vi "Bank With Semaphore.vi"() -> ()   [LabVIEW 2010]
doc: "This VI is a solution to the exercise in LabVIEW Core I that demonstrates race conditions. Without protecting critical code, as done here with semaphores, this VI could lose either a withdrawal or a deposit if done simultaneously."
panel:
  out "Balance":dbl
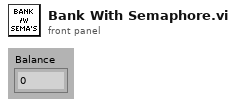
[diagram p1: front panel]
types:
  T1 = typedef "Account Info.ctl" = cluster{"Bank Rendezvous":T2, "Withdrawal Queue":refnum<queue>, "Deposit Queue":refnum<queue>}
  T2 = typedef "Rendezvous RefNum" = refnum<k1>
  T3 = typedef "Semaphore RefNum" = refnum<k1>
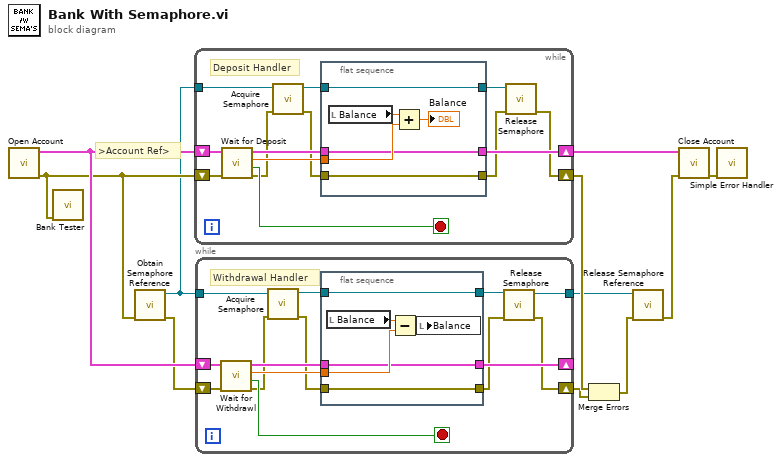
[diagram p0: block diagram]
diagram:
  # ">Account Ref>"
  n1 = call "Open Account.vi"() -> ("error out"=w6:errorcluster, "Account info"=w11:T1)  [unwired: 10 in]
  n2 = call "Bank Tester.vi"("error in (no error)"=w6) -> ()  [unwired: 10 in, 1 out]
  n3 = call <vilib>:"Obtain Semaphore Reference.vi"("error in (no error)"=w6) -> ("error out"=w5:errorcluster, "semaphore"=w1:T3)  [unwired: 4 in, 1 out]
  n4 = while {
    shift-right: [w20] -> w8
    shift-left: w11 -> [w23]
    shift-right: [w12] -> w10
    shift-left: w6 -> [w22]
    tunnel: w1 -> [w16]
    stop <- w19 stop-if-true
    # "Deposit Handler"
    n5 = call "Wait for Deposit.vi"("error in (no error)"=w22, "Account info"=w23) -> ("error out"=w15:errorcluster, "Stop?"=w19:bool, "Deposit Amount"=w24:dbl, "Account info out"=w21:T1)  [unwired: 6 in]
    n6 = call <vilib>:"Acquire Semaphore.vi"("error in (no error)"=w15, "semaphore"=w16) -> ("error out"=w14:errorcluster, "semaphore out"=w17:T3)  [unwired: 3 in, 1 out]
    n7 = flat-sequence {
      tunnel: w24 -> [w30]
      tunnel: [w27] -> w20
      tunnel: w21 -> [w27]
      tunnel: w14 -> [w26]
      tunnel: [w26] -> w13
      tunnel: [w25] -> w18
      tunnel: w17 -> [w25]
      frame #0 {
        n8 = local read "Balance"() -> (w28:dbl)
        n9 = Add(x=w28, y=w30) -> (x+y=→"Balance":dbl)
      }
    }
    n10 = call <vilib>:"Release Semaphore.vi"("error in (no error)"=w13, "semaphore"=w18) -> ("error out"=w12:errorcluster)  [unwired: 4 in, 1 out]
  }
  n11 = while {
    shift-right: [w40] -> _
    shift-left: w11 -> [w43]
    shift-right: [w31] -> w9
    shift-left: w5 -> [w42]
    tunnel: w1 -> [w38]
    tunnel: [w35] -> w4
    stop <- w39 stop-if-true
    # "Withdrawal Handler"
    n12 = call "Wait for Withdrawl.vi"("error in (no error)"=w42, "Account info"=w43) -> ("error out"=w34:errorcluster, "Stop?"=w39:bool, "Withdrawal Amount"=w44:dbl, "Account info out"=w41:T1)  [unwired: 6 in]
    n13 = call <vilib>:"Acquire Semaphore.vi"("error in (no error)"=w34, "semaphore"=w38) -> ("error out"=w33:errorcluster, "semaphore out"=w37:T3)  [unwired: 3 in, 1 out]
    n14 = flat-sequence {
      tunnel: w44 -> [w48]
      tunnel: w41 -> [w47]
      tunnel: w33 -> [w46]
      tunnel: [w47] -> w40
      tunnel: [w46] -> w32
      tunnel: w37 -> [w45]
      tunnel: [w45] -> w36
      frame #0 {
        n15 = local read "Balance"() -> (w49:dbl)
        n16 = Subtract(x=w49, y=w48) -> (x-y=w50:dbl)
        n17 = local write "Balance"(w50) -> ()
      }
    }
    n18 = call <vilib>:"Release Semaphore.vi"("error in (no error)"=w32, "semaphore"=w36) -> ("error out"=w31:errorcluster, "semaphore out"=w35:T3)  [unwired: 4 in]
  }
  n19 = Merge Errors(w10, w9) -> (w3:errorcluster)
  n20 = call <vilib>:"Release Semaphore Reference.vi"("error in (no error)"=w3, "semaphore"=w4) -> ("error out"=w2:errorcluster)  [unwired: 8 in, 1 out]
  n21 = call "Close Account.vi"("error in"=w2, "Account info"=w8) -> ("error out"=w7:errorcluster)  [unwired: 9 in]
  n22 = call <vilib>:"Simple Error Handler.vi"("error in (no error)"=w7) -> ()  [unwired: 4 in, 5 out]
